vi "NewTCS3472Sensor.vi"(8 "error in (no error)":errorcluster, 10 "I2C Slave Addr (0x29)":u8=41 format="%.0x", 11 "LINX I2C":refnum<class "LINX I2C.lvclass">) -> (0 "error out":errorcluster, 3 "TCS3472 out":refnum<class "TCS3472.lvclass">)   [LabVIEW 2020, in "TCS3472.lvclass"]
uses:
  TCS3472.lvclass
  LINX I2C/LINX I2C.lvclass
  TCS3472.lvclass/TCS3472.ctl
  Properties/Write LINX I2C.vi
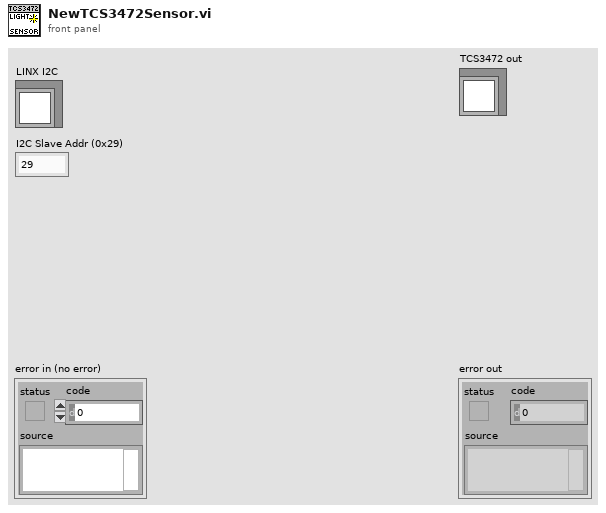
[diagram p1: front panel]
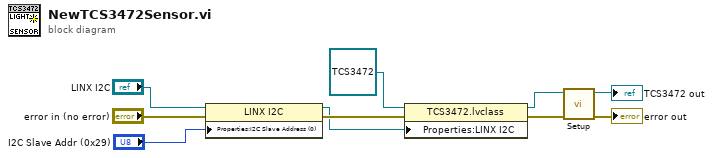
[diagram p0: block diagram]
diagram:
  n1 = property class="LINX I2C"(reference="LINX I2C", error in="error in (no error)", "Properties:I2C Slave Address (0)"="I2C Slave Addr (0x29)") -> (reference out=w4:refnum<class "LINX I2C.lvclass">, error out=w9:errorcluster)
  n2 = property class="TCS3472.lvclass"(reference=refnum<class "TCS3472.lvclass"> refnum ("TCS3472 out"), error in=w9, "Properties:LINX I2C"=w4) -> (reference out=w2:refnum<class "TCS3472.lvclass">, error out=w6:errorcluster)
  n3 = call "Setup.vi"("error in (no error)"=w6, "TCS3472 in"=w2) -> ("error out"=→"error out":errorcluster, "TCS3472 out"=→"TCS3472 out":refnum<class "TCS3472.lvclass">)  [unwired: 8 in]
